vi "Export Data.vi"(8 "error in (no error)":errorcluster, 11 "Graph Data":T1) -> (0 "error out":errorcluster)   [LabVIEW 2023]
doc: "Exports the currently displayed data and analysis to a tab separated text file suitable for loading in a spreadsheet application."
uses:
  controls/Graph Data.ctl
  <vilib>/Utility/miscctls.llb/LVAnnotationListTypeDef.ctl
  <vilib>/Utility/miscctls.llb/LVCursorListTypeDef.ctl
  <vilib>/Waveform/WDTFileIO.llb/Export Waveforms To Spreadsheet File (1D).vi
panel:
  # "(Scroll up to see large data cluster)"
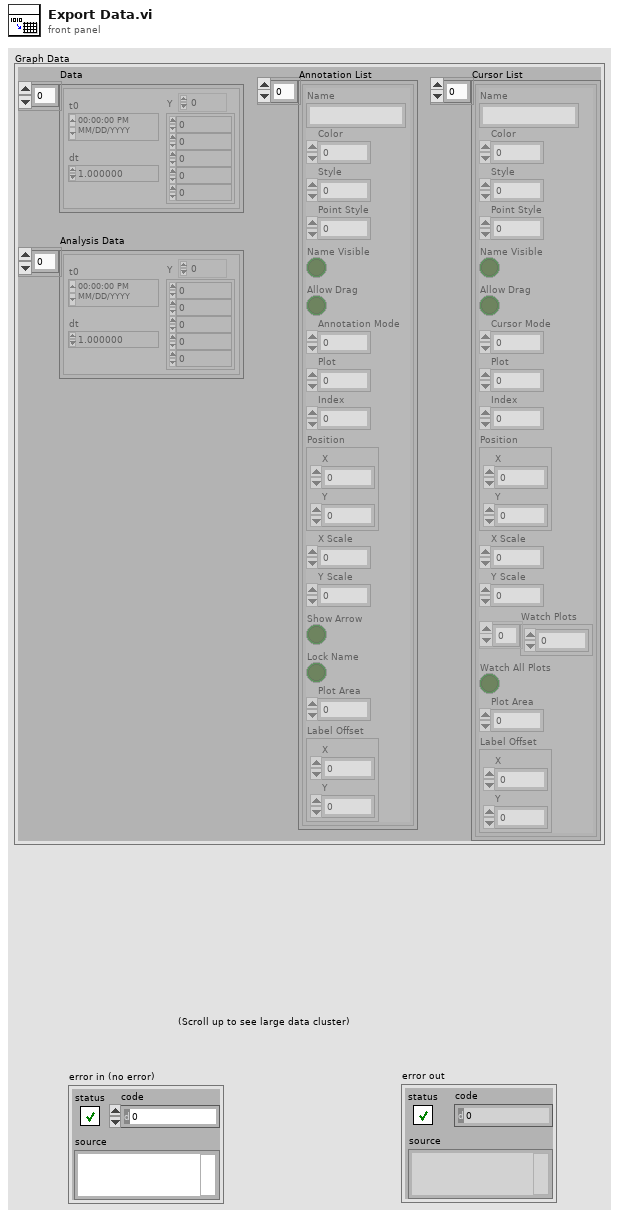
[diagram p1: front panel]
types:
  T1 = typedef "Graph Data.ctl" = cluster{"Data":waveform(dbl)[], "Annotation List":T2, "Cursor List":T3, "Analysis Data":waveform(dbl)[]}
  T2 = typedef "LVAnnotationListTypeDef.ctl" = cluster{"Name":string, "Color":u32, "Style":u8, "Point Style":u8, "Name Visible":bool, "Allow Drag":bool, "Annotation Mode":u32, "Plot":i32, "Index":i32, "Position":cluster{"X":dbl, "Y":dbl}, "X Scale":u32, "Y Scale":u32, "Show Arrow":bool, "Lock Name":bool, "Plot Area":i32, "Label Offset":cluster{"X":dbl, "Y":dbl}}[]
  T3 = typedef "LVCursorListTypeDef.ctl" = cluster{"Name":string, "Color":u32, "Style":u8, "Point Style":u8, "Name Visible":bool, "Allow Drag":bool, "Cursor Mode":u32, "Plot":i32, "Index":i32, "Position":cluster{"X":dbl, "Y":dbl}, "X Scale":u32, "Y Scale":u32, "Watch Plots":i32[], "Watch All Plots":bool, "Plot Area":i32, "Label Offset":cluster{"X":dbl, "Y":dbl}}[]
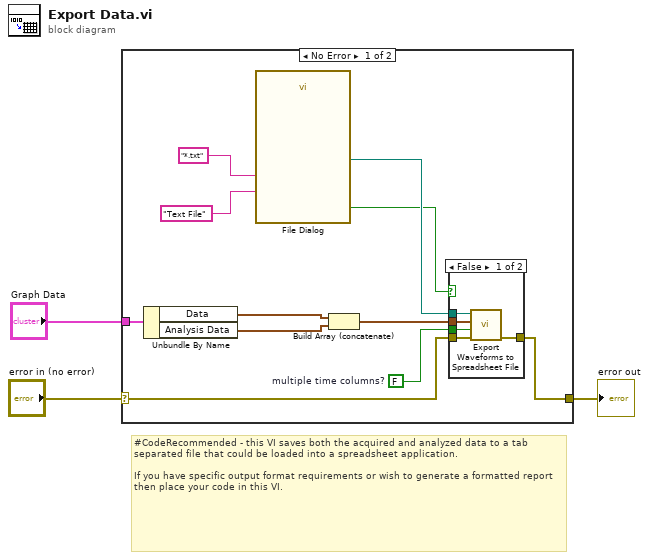
[diagram p0: block diagram]
diagram:
  # "#CodeRecommended - this VI saves both the acquired and analyzed data to a tab separated file that could be loaded into a spreadsheet application.\n\nIf you have specific output format requirements or wish to generate a formatted report then place your code in this VI."
  n1 = case shown="No Error" "error in (no error)" {
    selector: "error in (no error)" -> [w12 w21]
    tunnel: "Graph Data" -> [w14 _]
    tunnel: [w11 w21] -> w2
    frame No Error {
      w13 = FALSE  # multiple time columns?
      n2 = Unbundle By Name(w14) -> ("Data"=w10:waveform(dbl)[], "Analysis Data"=w9:waveform(dbl)[])
      n3 = call "File Dialog"("pattern (all files)"="*.txt", "pattern label"="Text File" ("Text File")) -> ("selected path"=w7:path, "cancelled"=w4:bool)  [unwired: 10 in, 2 out]
      n4 = Build Array (concatenate)(w10, w9) -> (w8:waveform(dbl)[])
      n5 = case shown="False" w4 {
        tunnel: w13 -> [w19 _]
        tunnel: w12 -> [w18 w20]
        tunnel: [w17 w20] -> w11
        tunnel: w8 -> [w16 _]
        tunnel: w7 -> [w15 _]
        frame False {
          n6 = call-poly <vilib>:"Export Waveforms to Spreadsheet File.vi"("error in (no error)"=w18, "multiple time columns? (single:F)"=w19, "waveforms"=w16, "file path (dialog if empty)"=w15) -> ("error out"=w17:errorcluster)  [unwired: 6 in, 1 out]
        }
        frame True {
        }
      }
    }
    frame Error {
    }
  }
  "error out" <- w2
